vi "Experiment.vi"() -> ()   [LabVIEW 2013]
uses:
  <vilib>/DAQmx/read.llb/DAQmx Read (Analog 1D Wfm NChan 1Samp).vi
  <vilib>/DAQmx/read.llb/DAQmx Read (Analog Wfm 1Chan 1Samp).vi
  <vilib>/DAQmx/miscellaneous.llb/DAQmx Fill In Error Info.vi
panel:
  out "RTD Temperature":waveform(dbl)(graph)
  out "Iteration":i32
  out "Shunt - Current":dbl(knob) scale=0.0..30.0
  out "Total":dbl(knob) scale=0.0..30.0
  out "Gray-Orange Resistor":dbl(knob) scale=0.0..30.0
  out "Orange-Red Resistor":dbl(knob) scale=0.0..30.0
  in  "stop 3":bool
  out "Red-Gray Resistor":dbl(knob) scale=0.0..30.0
  in  "stop":bool
  out "RTD":dbl(slide) scale=0.0..100.0
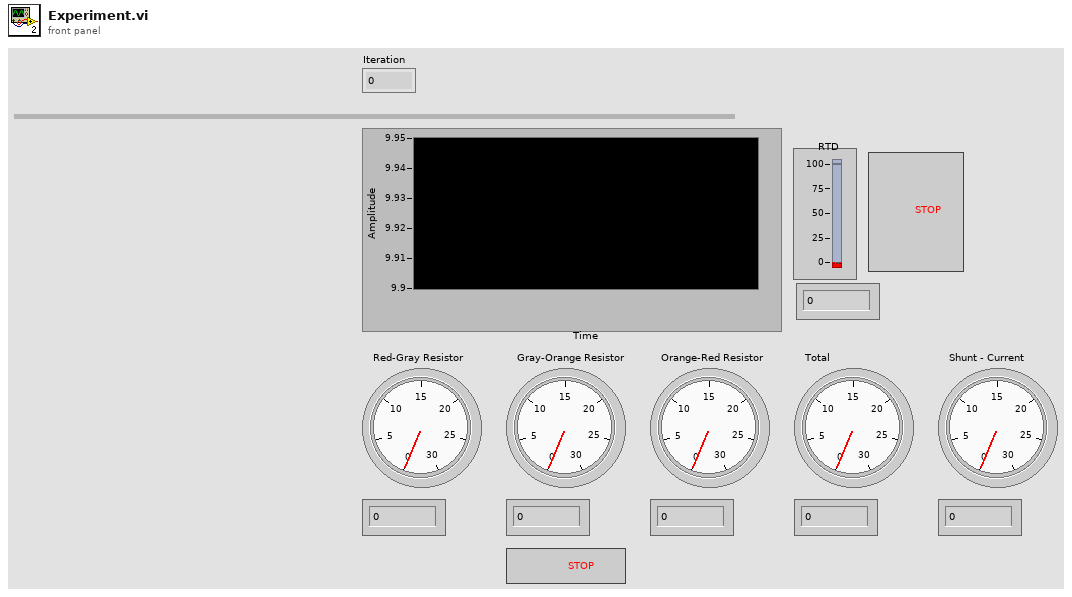
[diagram p1: front panel]
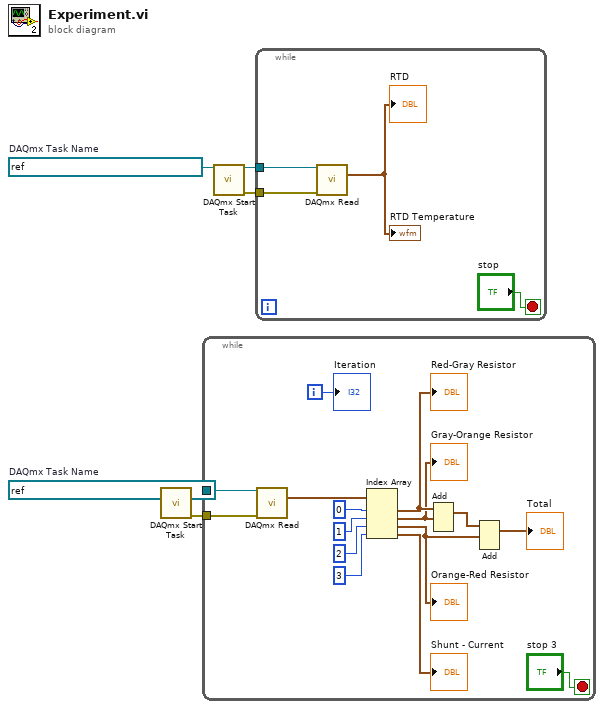
[diagram p0: block diagram]
diagram:
  w1 = refnum<k21> "Voltage and Current Reading Task"  # DAQmx Task Name
  w6 = refnum<k21> "RTD Temperature Reading Task"  # DAQmx Task Name
  n1 = call <vilib>:"DAQmx Start Task.vi"("task/channels in"=w1) -> ("task out"=w3:refnum<k21>, "error out"=w2:errorcluster)  [unwired: 13 in]
  n2 = while {
    tunnel: w3 -> [w20]
    tunnel: w2 -> [w19]
    i -> [w9]
    stop <- "stop 3" stop-if-true
    n3 = call-poly <vilib>:"DAQmx Read.vi"("task/channels in"=w20, "error in"=w19) -> ("data"=w7:waveform(dbl)[])  [unwired: 11 in, 2 out]
    n4 = Index Array(array=w7, index #1=0 ("index"), index #2=1 ("index"), index #3=2 ("index"), index #4=3 ("index")) -> (element #1=w15:waveform(dbl), element #2=w13:waveform(dbl), element #3=w11:waveform(dbl), element #4=→"Shunt - Current":waveform(dbl))
    "Red-Gray Resistor" <- w15
    "Orange-Red Resistor" <- w11
    "Gray-Orange Resistor" <- w13
    n5 = Add(1:w13, 2:w15) -> (0:w17:waveform(dbl))  [unwired: 1 in, 1 out]
    n6 = Add(1:w11, 2:w17) -> (0:→"Total":waveform(dbl))  [unwired: 1 in, 1 out]
    "Iteration" <- w9
  }
  n7 = call <vilib>:"DAQmx Start Task.vi"("task/channels in"=w6) -> ("task out"=w5:refnum<k21>, "error out"=w4:errorcluster)  [unwired: 13 in]
  n8 = while {
    tunnel: w5 -> [w24]
    tunnel: w4 -> [w23]
    stop <- "stop" stop-if-true
    n9 = call-poly <vilib>:"DAQmx Read.vi"("task/channels in"=w24, "error in"=w23) -> ("data"=→"RTD" →"RTD Temperature":waveform(dbl))  [unwired: 11 in, 2 out]
  }
